vi "LDO Modbus Setup Part 1.vi"(7 "Initialize?":bool, 8 "error in (no error)":errorcluster, 11 "Queue in":refnum<queue>) -> (0 "error out":errorcluster, 3 "dup Message Queue":refnum<queue>)   [LabVIEW 2020]
uses:
  Message Queue/Message Cluster.ctl
  Message Queue/Message Queue.lvlib
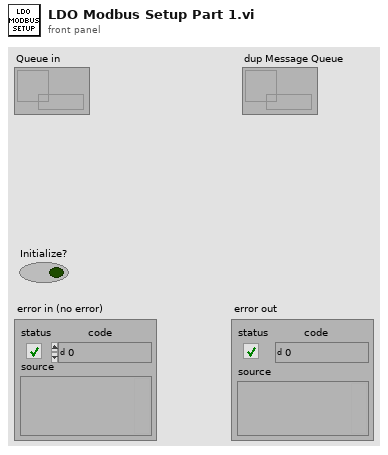
[diagram p1: front panel]
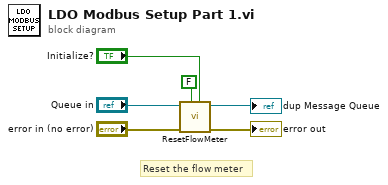
[diagram p0: block diagram]
diagram:
  # "Reset the flow meter"
  n1 = call "ResetFlowMeter.vi"("Initialize?"="Initialize?", "FVIR?"=FALSE, "error in (no error)"="error in (no error)", "Modbus Queue in"="Queue in") -> ("error out"=→"error out":errorcluster, "dup Message Queue"=→"dup Message Queue":refnum<queue>)  [unwired: 6 in]
